vi "FestoCPX.Station.ButtonLed.On.vi"(8 "error in":errorcluster, 10 "Button Led":T1, 11 "Blink period [ms] (0)":u32) -> (0 "error out":errorcluster)   [LabVIEW 2016]
uses:
  FestoCPX.Station.ButtonLed.ctl
  FestoCPX.Station.TowerLed.Fglb.Action.ctl
  FestoCPX.DO.Signal.ctl
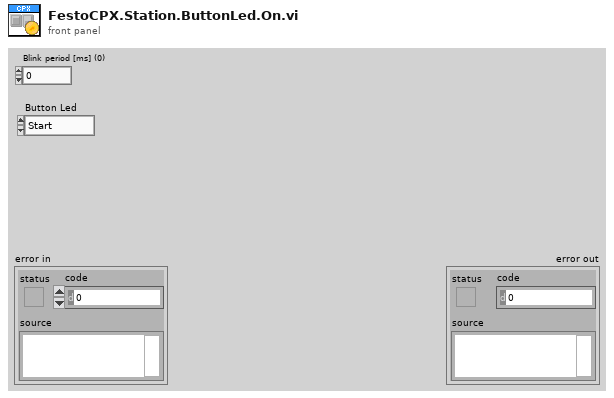
[diagram p1: front panel]
types:
  T1 = typedef "FestoCPX.Station.ButtonLed.ctl" = enum16{"Start", "Stop", "Control"}
  T2 = typedef "FestoCPX.Station.TowerLed.Fglb.Action.ctl" = enum16{"init", "set", "get"}
  T3 = typedef "FestoCPX.DO.Signal.ctl" = enum16{"Safety Reset", "Air Main Valve", "Door Lock", "Button LED Start", "Button LED Stop", "Button LED Control", "Traffic LED Red", "Traffic LED Orange", "Traffic LED Green", "Horn", "Laser Interlock", "Laser Trigger", "Laser Fume Extractor", "Product Suction Gripper Slot 1 A", "Product Suction Gripper Slot 1 B", "Product Suction Gripper Slot 2 A", "Product Suction Gripper Slot 2 B", "Product Suction Gripper Slot 3 A", "Product Suction Gripper Slot 3 B", "Product Suction Gripper Slot 4 A", "Product Suction Gripper Slot 4 B", "Product Suction Gripper Final A", "Product Suction Gripper Final B", "Lamp", "Q1 Product Move Work", "Q1 Product Move Home", "Q2 Table Turn Work", "Q2 Table Turn Home", "Q3 Product Lift A", "Q3 Product Lift B", "Q4 Product Arm OK", "Q4 Product Arm NOK", "Q5 Product Arm Work", "Q6 Product BlowOut A", "Q6 Product BlowOut B"}
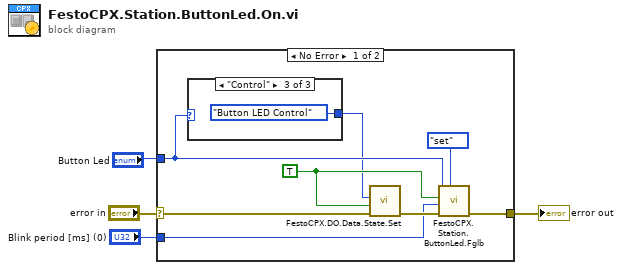
[diagram p0: block diagram]
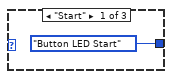
[diagram p2: hidden frame]
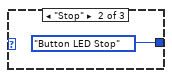
[diagram p3: hidden frame]
diagram:
  n1 = case shown="No Error" "error in" {
    selector: "error in" -> [w12 w16]
    tunnel: [w9 w16] -> w4
    tunnel: "Button Led" -> [w6 _]
    tunnel: "Blink period [ms] (0)" -> [w7 _]
    frame No Error {
      w8 = TRUE ("State")
      n2 = case shown="\"Control\"" w6 {
        tunnel: [FestoCPX.DO.Signal."Button LED Start" ("DI Signal") FestoCPX.DO.Signal."Button LED Stop" ("DI Signal") FestoCPX.DO.Signal."Button LED Control" ("DI Signal")] -> w5
        frame "Start" {
        }
        frame "Stop" {
        }
        frame "Control" {
        }
      }
      n3 = call "FestoCPX.DO.Data.State.Set.vi"("error in (no error)"=w12, "State"=w8, "CPX.DO"=w5) -> ("error out"=w10:errorcluster)  [unwired: 8 in]
      n4 = call "FestoCPX.Station.ButtonLed.Fglb.vi"("Action (get)"=FestoCPX.Station.TowerLed.Fglb.Action."set", "error in"=w10, "Blink period [ms] (0)"=w7, "State"=w8, "ButtonLed"=w6) -> ("error out"=w9:errorcluster)  [unwired: 4 in, 2 out]
    }
    frame Error {
    }
  }
  "error out" <- w4
